vi "Flight Gear Interface RT Driver VI.vi"(6 "Device Clock":string, 9 "Device Inputs FIFO":refnum<k33>, 11 "Device Reference":T1 format="%.0x") -> ()   [LabVIEW 2010, in "Flight Gear Interface Custom Device.lvlib"]
uses:
  Flight Gear Interface Custom Device.lvlib
  <vilib>/NI VeriStand/Custom Device API/Custom Device Item Ref.ctl
  <vilib>/NI VeriStand/Custom Device API/Custom Device Channel Type.ctl
  FlightGearState.ctl
  FGNetFDM.ctl
  <vilib>/Platform/TimedLoop/XDataNode/XDataNode.xnode
  <vilib>/Platform/TimedLoop/XDataNode/timing_clust.ctl
  <vilib>/Platform/TimedLoop/XDataNode/nitl_modes.ctl
  <vilib>/Platform/TimedLoop/XDataNode/wakeup.ctl
  <vilib>/NI VeriStand/Custom Device API/Get Item Property (U16).vi
  <vilib>/NI VeriStand/Custom Device API/Get Item Property (I32).vi
  <vilib>/NI VeriStand/Custom Device API/Get Item Property (String).vi
  <vilib>/Platform/TimedLoop/XDataNode/XDNodeRunTimeDep.lvlib
  <vilib>/NI Veristand/Custom Device API/Custom Device API.lvlib
  <vilib>/NI Veristand/Custom Device Tools/Custom Device Utility Library/Custom Device Utility Library.lvlib
panel:
  in  "Status Notifier":refnum<notifier>
  # "Custom Device Template\nv1.0"
  # "Use this template as a starting point for creating a custom device code module. The input controls shown here are specially named controls that the system will use to provide the device loop with data. The controls are not required for the device loop to run. For instance, if the device doesn't produce any output data, then you don't need the Device Outputs FIFO control. If you do use these controls, however, they need to have these exact names to be functional."
  # "The optional status notifier element is used to notify the RT engine of the last state of the custom device, and to indicate the device has completed execution. If this control is not used, a default No Error value is returned to the system when the device finishes execution.\n\nNote: This error state is not checked until the system shuts down. Use an output status channel to send more immediate status values to the system."
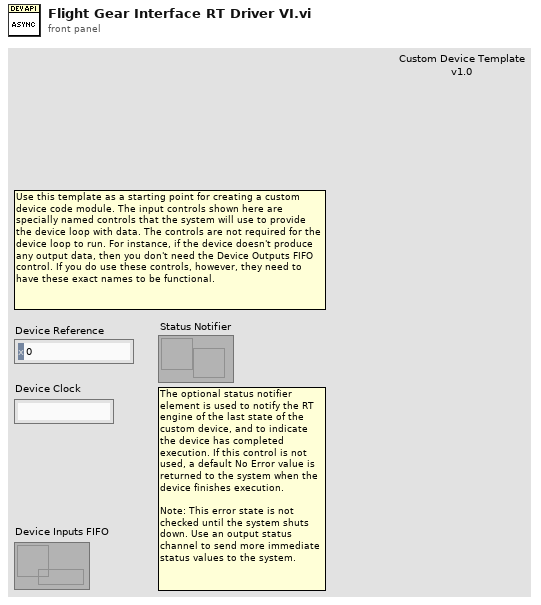
[diagram p1: front panel]
types:
  T1 = typedef "Custom Device API.lvlib/Custom Device Item Ref.ctl" = u64
  T2 = typedef "Flight Gear Interface Custom Device.lvlib/FGNetFDM.ctl" = cluster{"Version":cluster{"version":u32, "pad":u32}, "Positions":cluster{"Doubles":cluster{"longitude":dbl, "latitude":dbl, "altitude":dbl}, "Singles":cluster{"agl":sgl, "phi":sgl, "theta":sgl, "psi":sgl, "alpha":sgl, "beta":sgl}}, "Velocities":cluster{"phidot":sgl, "thetadot":sgl, "psidot":sgl, "vcas":sgl, "climb_rate":sgl, "v_north":sgl, "v_east":sgl, "v_down":sgl, "v_wind_body_north":sgl, "v_wind_body_east":sgl, "v_wind_body_down":sgl}, "Accelerations":cluster{"A_X_pilot":sgl, "A_Y_pilot":sgl, "A_Z_pilot":sgl}, "Stall":cluster{"stall_warning":sgl, "slip_deg":sgl}, "Engine Status":cluster{"num_engines":u32, "eng_state":u32[], "rpm":sgl[], "fuel_flow":sgl[], "fuel_px":sgl[], "egt":sgl[], "cht":sgl[], "mp_osi":sgl[], "tit":sgl[], "oil_temp":sgl[], "oil_px":sgl[]}, "Consumables":cluster{"num_tanks":u32, "fuel_quantity":sgl[]}, "Gear Status":cluster{"num_wheels":u32, "wow":u32[], "gear_pos":sgl[], "gear_steer":sgl[], "gear_compression":sgl[]}, "Environment":cluster{"curr_time":u32, "warp":i32, "visibility":sgl}, "Control Surface Positions":cluster{"elevator":sgl, "elevator_trim_tab":sgl, "left_flap":sgl, "right_flap":sgl, "left aileron":sgl, "right_aileron":sgl, "rudder":sgl, "nose_wheel":sgl, "speedbrake":sgl, "spoilers":sgl}}
  T3 = typedef "Flight Gear Interface Custom Device.lvlib/FlightGearState.ctl" = enum16{"Initialize", "Write", "Close"}
  T4 = typedef "Custom Device API.lvlib/Custom Device Channel Type.ctl" = enum16{"Input", "Output"}
  T5 = typedef "Custom Device API.lvlib/Custom Device Timed Loop Priority.ctl" = enum32{"Low", "Medium", "High"}
  T6 = typedef "XDNodeRunTimeDep.lvlib/timing_clust.ctl" = cluster{"Expected End [f-1]":u64, "Actual End [f-1]":u64, "Finished Late? [f-1]":bool, "Expected End [i-1]":u64, "Actual End [i-1]":u64, "Finished Late? [i-1]":bool, "Expected Start [i]":u64, "Actual Start [i]":u64, "Expected Start [f]":u64, "Actual Start [f]":u64, "Source Name":string, "Structure Name":string, "Period":i64, "Deadline":i64, "Offset":i64, "Start":i64, "Priority":i32, "Timeout":i32, "Mode":T7, "Wakeup Reason":T8, "Error":errorcluster, "Source Type":string, "Secondary Source Type":string, "Global End Time":u64, "Global Start Time":u64, "Frame Duration":u64, "Iteration Duration":u64, "Assigned CPU":i32, "I/O Scan Engine Mode":u32}
  T7 = typedef "XDNodeRunTimeDep.lvlib/nitl_modes.ctl" = enum32{"No Change", "Process missed periods, maintain original phase", "Discard missed periods, maintain original phase", "Process missed periods, ignore original phase", "Discard missed periods, ignore original phase"}
  T8 = typedef "XDNodeRunTimeDep.lvlib/wakeup.ctl" = enum32{"Normal", "Aborted", "Asynchronous wakeup", "Timing source error", "Timed loop error", "Timeout"}
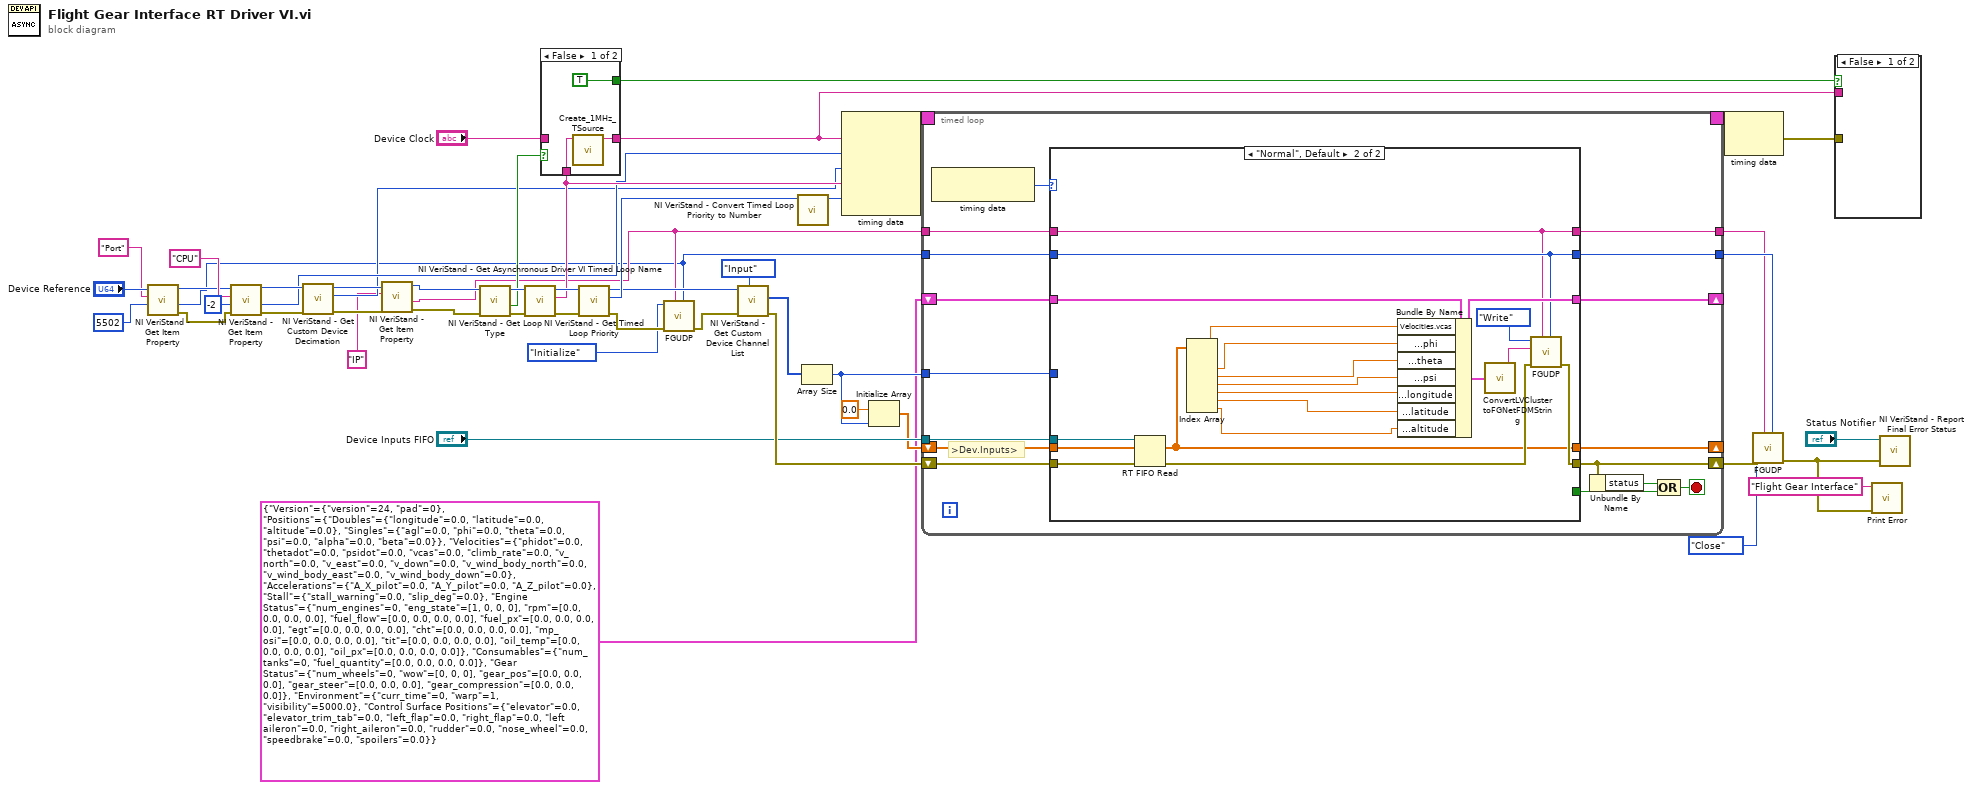
[diagram p0: block diagram]
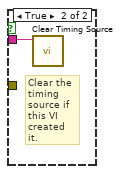
[diagram p2: hidden frame]
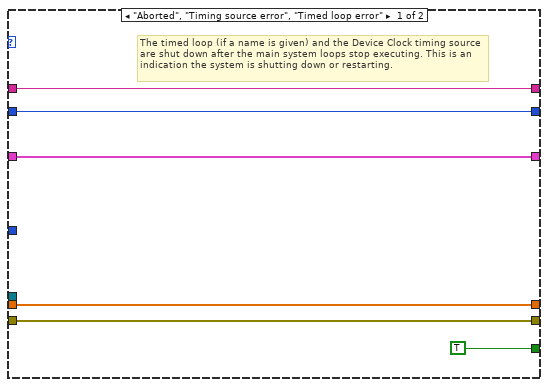
[diagram p4: hidden frame]
diagram:
  n1 = call-poly <vilib>:"NI VeriStand - Get Item Property.vi"("Default Value"=u16 5502 ("Remote Port"), "Property Name"="Port", "Item Ref in"="Device Reference") -> ("error out"=w7:errorcluster, "Value"=w3:u16, "Item Ref out"=w8:T1)  [unwired: 5 in, 1 out]
  n2 = call-poly <vilib>:"NI VeriStand - Get Item Property.vi"("error in (no error)"=w7, "Default Value"=-2, "Property Name"="CPU", "Item Ref in"=w8) -> ("error out"=w17:errorcluster, "Value"=w15:i32, "Item Ref out"=w18:T1)  [unwired: 4 in, 1 out]
  n3 = call <vilib>:"NI VeriStand - Get Custom Device Decimation.vi"("error in (no error)"=w17, "Device Ref in"=w18) -> ("error out"=w21:errorcluster, "Decimation"=w13:i32, "Device Ref out"=w20:T1)  [unwired: 7 in]
  n4 = call-poly <vilib>:"NI VeriStand - Get Item Property.vi"("error in (no error)"=w21, "Property Name"="IP", "Item Ref in"=w20) -> ("error out"=w14:errorcluster, "Value"=w11:string, "Item Ref out"=w19:T1)  [unwired: 5 in, 1 out]
  n5 = call <vilib>:"NI VeriStand - Get Loop Type.vi"("error in (no error)"=w14, "Device Ref in"=w19) -> ("error out"=w38:errorcluster, "Use Device Clock"=w36:bool, "Device Ref out"=w37:T1)  [unwired: 7 out]
  n6 = call <vilib>:"NI VeriStand - Get Asynchronous Driver VI Timed Loop Name.vi"("error in (no error)"=w38, "Device Ref in"=w37) -> ("error out"=w43:errorcluster, "Device Timed Loop Name"=w30:string, "Device Ref out"=w50:T1)  [unwired: 7 out]
  n7 = case shown="False" w36 {
    tunnel: "Device Clock" -> [_ w55]
    tunnel: [w54 w55] -> w31
    tunnel: [TRUE _] -> w32
    tunnel: w30 -> [w52 _]
    frame False {
      n8 = call <vilib>:"Create_1MHz_TSource.vi"("name (in)"=w52) -> ("name (out)"=w54:string)  [unwired: 9 in, 1 out]
    }
    frame True {
    }
  }
  n9 = call <vilib>:"NI VeriStand - Get Timed Loop Priority.vi"("error in (no error)"=w43, "Device Ref in"=w50) -> ("error out"=w28:errorcluster, "Priority"=w41:T5, "Device Ref out"=w29:T1)  [unwired: 7 out]
  n10 = call "FGUDP.vi"("Remote Port"=w3, "Remote Host"=w11, "Error In"=w28, "UDP State"=FlightGearState."Initialize") -> ("error out"=w27:errorcluster)  [unwired: 7 in]
  n11 = call <vilib>:"NI VeriStand - Get Custom Device Channel List.vi"("Channel Type"=Custom_Device_Channel_Type."Input", "error in (no error)"=w27, "Device Ref in"=w29) -> ("error out"=w51:errorcluster, "Specified Channel Ref List"=w42:T1[])  [unwired: 7 out]
  n12 = call <vilib>:"NI VeriStand - Convert Timed Loop Priority to Number.vi"("Priority"=w41) -> ("Numeric Priority"=w40:i32)  [unwired: 10 out]
  n13 = Array Size(array=w42) -> (size(s)=w39:i32)
  n14 = node-c288(w31, w15, w13, w30, w40) -> (w48:T6)
  n15 = Initialize Array(0.0 ("element"), w39) -> (w45:dbl[])
  n16 = timed-loop {
    timing: w48 -> [_]
    timing-out: [_] -> w47
    shift-right: [w69] -> _
    shift-left: w45 -> [w70]
    shift-right: [w66] -> w25
    shift-left: w51 -> [w71]
    tunnel: "Device Inputs FIFO" -> [w67]
    tunnel: w39 -> [w62]
    shift-right: [w59] -> _
    shift-left: T2 {"Version"={"version"=24, "pad"=0}, "Positions"={"Doubles"={"longitude"=0.0, "latitude"=0.0, "altitude"=0.0}, "Singles"={"agl"=0.0, "phi"=0.0, "theta"=0.0, "psi"=0.0, "alpha"=0.0, "beta"=0.0}}, "Velocities"={"phidot"=0.0, "thetadot"=0.0, "psidot"=0.0, "vcas"=0.0, "climb_rate"=0.0, "v_north"=0.0, "v_east"=0.0, "v_down"=0.0, "v_wind_body_north"=0.0, "v_wind_body_east"=0.0, "v_wind_body_down"=0.0}, "Accelerations"={"A_X_pilot"=0.0, "A_Y_pilot"=0.0, "A_Z_pilot"=0.0}, "Stall"={"stall_warning"=0.0, "slip_deg"=0.0}, "Engine Status"={"num_engines"=0, "eng_state"=[1, 0, 0, 0], "rpm"=[0.0, 0.0, 0.0, 0.0], "fuel_flow"=[0.0, 0.0, 0.0, 0.0], "fuel_px"=[0.0, 0.0, 0.0, 0.0], "egt"=[0.0, 0.0, 0.0, 0.0], "cht"=[0.0, 0.0, 0.0, 0.0], "mp_osi"=[0.0, 0.0, 0.0, 0.0], "tit"=[0.0, 0.0, 0.0, 0.0], "oil_temp"=[0.0, 0.0, 0.0, 0.0], "oil_px"=[0.0, 0.0, 0.0, 0.0]}, "Consumables"={"num_tanks"=0, "fuel_quantity"=[0.0, 0.0, 0.0, 0.0]}, "Gear Status"={"num_wheels"=0, "wow"=[0, 0, 0], "gear_pos"=[0.0, 0.0, 0.0], "gear_steer"=[0.0, 0.0, 0.0], "gear_compression"=[0.0, 0.0, 0.0]}, "Environment"={"curr_time"=0, "warp"=1, "visibility"=5000.0}, "Control Surface Positions"={"elevator"=0.0, "elevator_trim_tab"=0.0, "left_flap"=0.0, "right_flap"=0.0, "left aileron"=0.0, "right_aileron"=0.0, "rudder"=0.0, "nose_wheel"=0.0, "speedbrake"=0.0, "spoilers"=0.0}} ("Cluster") -> [w61]
    tunnel: w3 -> [w60]
    tunnel: [w58] -> w23
    tunnel: w11 -> [w57]
    tunnel: [w56] -> w22
    stop <- w63 stop-if-true
    # ">Dev.Inputs>"
    n17 = node-c288() -> (w68:T8)  [unwired: 1 out]
    n18 = case shown="\"Normal\", Default" w68 {
      tunnel: w71 -> [w76 w94]
      tunnel: w70 -> [w77 w95]
      tunnel: [w76 w92] -> w66
      tunnel: [w77 w91] -> w69
      tunnel: w67 -> [_ w96]
      tunnel: [TRUE _] -> w64
      tunnel: w62 -> [_ _]
      tunnel: w61 -> [w74 w90]
      tunnel: w60 -> [w73 w82]
      tunnel: [w74 w83] -> w59
      tunnel: [w73 w82] -> w58
      tunnel: w57 -> [w72 w81]
      tunnel: [w72 w81] -> w56
      frame "Aborted", "Timing source error", "Timed loop error" {
        # "The timed loop (if a name is given) and the Device Clock timing source are shut down after the main system loops stop executing. This is an indication the system is shutting down or restarting."
      }
      frame "Normal", Default {
        n19 = RT FIFO Read(0:w96, 1:w95, 3:w94) -> (9:w91:dbl[], 11:w93:errorcluster)  [unwired: 4 out]
        n20 = Index Array(array=w91) -> (element #1=w88:dbl, element #2=w89:dbl, element #3=w87:dbl, element #4=w86:dbl, element #5=w78:dbl, element #6=w80:dbl, element #7=w79:dbl)  [unwired: 7 in]
        n21 = Bundle By Name(cluster=w90, "Velocities.vcas"=w88, "Positions.Singles.phi"=w89, "Positions.Singles.theta"=w87, "Positions.Singles.psi"=w86, "Positions.Doubles.longitude"=w78, "Positions.Doubles.latitude"=w80, "Positions.Doubles.altitude"=w79) -> (w83:T2)
        n22 = call "ConvertLVClustertoFGNetFDMString.vi"("Cluster"=w83) -> ("FGNetFDM"=w85:string)
        n23 = call "FGUDP.vi"("Remote Port"=w82, "Remote Host"=w81, "Error In"=w93, "Data String"=w85, "UDP State"=FlightGearState."Write") -> ("error out"=w92:errorcluster)  [unwired: 6 in]
      }
    }
    n24 = Unbundle By Name(w66) -> ("status"=w65:bool)
    n25 = Compound Arithmetic op=OR(w65, w64) -> (w63:bool)
  }
  n26 = node-c288(w47) -> (w33:errorcluster)
  n27 = call "FGUDP.vi"("Remote Port"=w23, "Remote Host"=w22, "Error In"=w25, "UDP State"=FlightGearState."Close") -> ("error out"=w2:errorcluster)  [unwired: 7 in]
  n28 = case shown="False" w32 {
    tunnel: w33 -> [_ _]
    tunnel: w31 -> [_ w100]
    frame False {
    }
    frame True {
      # "Clear the timing source if this VI created it."
      n29 = call <vilib>:"Clear Timing Source.vi"("name"=w100) -> ()  [unwired: 1 in, 10 out]
    }
  }
  n30 = call "Print Error.vi"("error out"=w2, "Your code's public name"="Flight Gear Interface") -> ()  [unwired: 9 in]
  n31 = call <vilib>:"NI VeriStand - Report Final Error Status.vi"("error in (no error)"=w2, "Status Notifier"="Status Notifier") -> ()  [unwired: 1 in, 9 out]
